vi "RP proccess data.vi"() -> ()   [LabVIEW 2015]
uses:
  <vilib>/Analysis/NI_AALPro.lvlib
panel:
  in  "Filed tiime shift":dbl format="%#_6p"
  out "Phase":dbl
  out "Waveform Graph 2":waveform(dbl)(graph)
  in  "Clip units of Ts off":dbl
  in  "Filter type":enum16{"None", "IIR", "FIR"}(ring)=enum."FIR"
  in  "Save output":bool
  in  "Phase shift":dbl step=90.0
  in  "Integrate Bdot":bool
  in  "Fix time delay":bool=TRUE
  in  "Time constant":dbl=0.0001 format="%#_6p"
  out "XY Graph":cluster{dbl[], "Y":dbl[]}[](graph)
  out "Error Out":errorcluster
  in  "Bdot calibration":dbl=2506.0
  in  "offset length":i32=990000
  out "Waveform Graph":waveform(dbl)[](graph)
  in  "Bdot channel":string="Field_fixed"
  in  "Signal channel":string="CH0"
  in  "Bdot file":path
  in  "Signal file":path
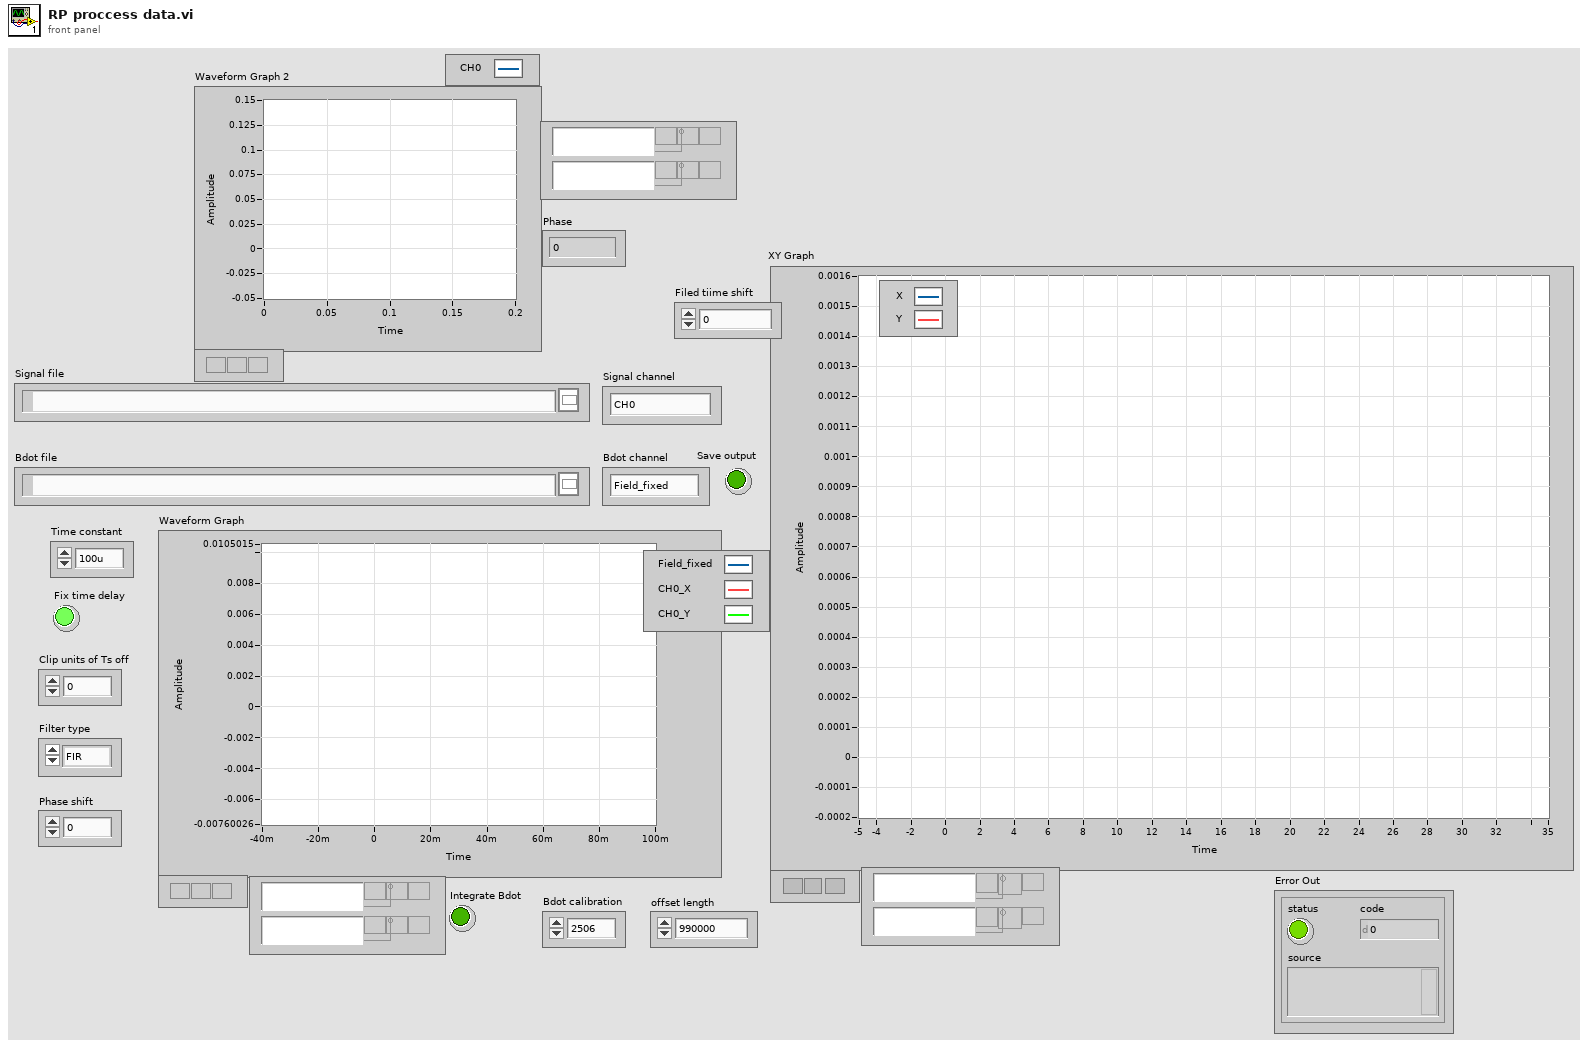
[diagram p1: front panel]
types:
  T1 = enum16{"open", "open or create", "create or replace", "create", "open (read-only)"}
  T2 = cluster{"Waveform":waveform(dbl), "Waveform":waveform(dbl)}
  T3 = cluster{"Waveform":waveform(dbl), "Waveform":waveform(dbl)}[]
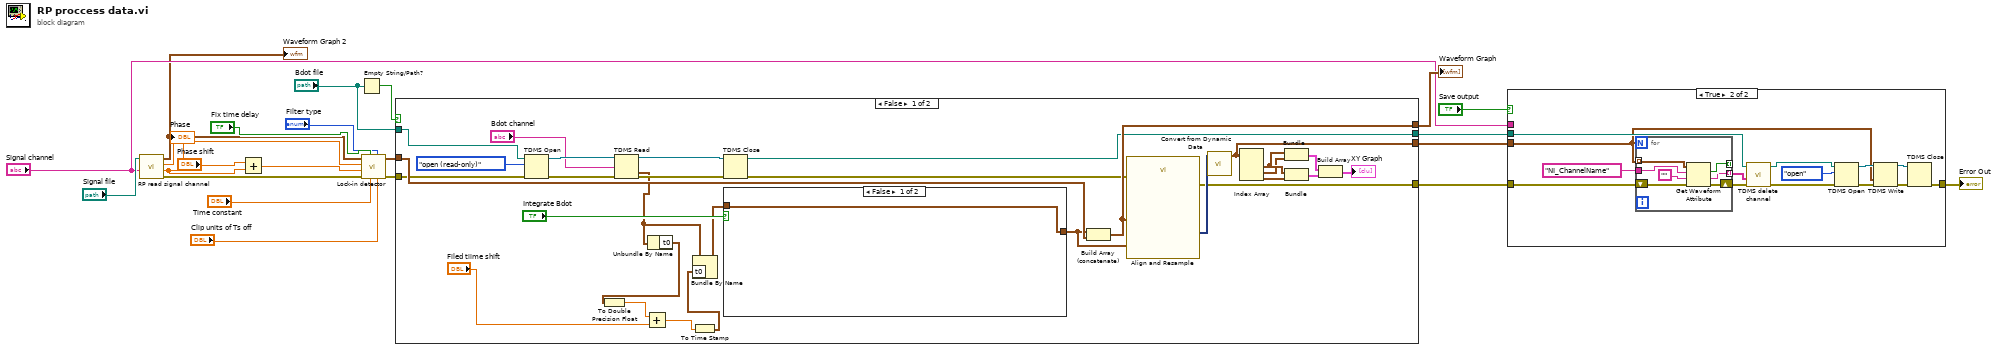
[diagram p0: block diagram]
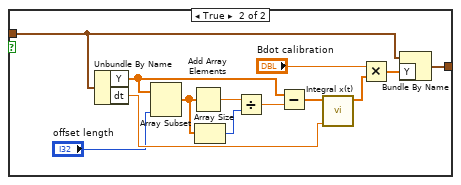
[diagram p2: hidden frame]
diagram:
  n1 = call "RP read signal channel.vi"("Channel name"="Signal channel", "File"="Signal file") -> ("Error Out"=w19:errorcluster, "Phase"=w20:dbl, "Frequency"=w21:dbl, "Data out"=w1:waveform(dbl))  [unwired: 3 in, 3 out]
  "Waveform Graph 2" <- w1
  "Phase" <- w20
  n2 = Add(x="Phase shift", y=w20) -> (x+y=w14:dbl)
  n3 = Empty String/Path?(string/path="Bdot file") -> (empty?=w4:bool)
  n4 = call "Lock-in detector.vi"("Clip units of Ts off"="Clip units of Ts off", "Filter type"="Filter type", "Time constant"="Time constant", "Fix time delay"="Fix time delay", "Error In"=w19, "Phase"=w14, "Frequency"=w21, "Data in"=w1) -> ("Error Out"=w3:errorcluster, "Data out"=w16:waveform(dbl)[])  [unwired: 2 in]
  n5 = case shown="False" w4 {
    tunnel: w16 -> [w45 w69]
    tunnel: [w38 w69] -> w15
    tunnel: [w37 w68] -> w11
    tunnel: [w34 w69] -> w8
    tunnel: "Bdot file" -> [w33 w68]
    tunnel: w3 -> [w30 w67]
    tunnel: [w31 w67] -> w2
    frame False {
      n6 = TDMS Open(8:w30, 10:T1."open (read-only)" ("operation (0:open)"), 11:w33) -> (0:w51:errorcluster, 3:w50:refnum<k34>)  [unwired: 4 in]
      n7 = TDMS Read(0:w50, 7:"Bdot channel", 11:w51) -> (4:w47:refnum<k34>, 10:w24:waveform(dbl), 15:w48:errorcluster)  [unwired: 5 in, 3 out]
      n8 = Unbundle By Name(w24) -> ("t0"=w29:timestamp)
      n9 = To Double Precision Float(number=w29) -> (double precision float=w28:dbl)
      n10 = Add(x=w28, y="Filed tiime shift") -> (x+y=w26:dbl)
      n11 = To Time Stamp(1:w26) -> (0:w25:timestamp)
      n12 = Bundle By Name(cluster=w24, "t0"=w25) -> (w23:waveform(dbl))
      n13 = TDMS Close(8:w48, 11:w47) -> (0:w32:errorcluster, 3:w37:path)
      n14 = case shown="False" "Integrate Bdot" {
        tunnel: w23 -> [w53 w56]
        tunnel: [w53 w54] -> w44
        frame False {
        }
        frame True {
          n15 = Unbundle By Name(w56) -> ("Y"=w59:dbl[], "dt"=w66:dbl)
          n16 = Array Subset(array=w59, length="offset length") -> (w63:dbl[])  [unwired: 1 in]
          n17 = Add Array Elements(numeric array=w63) -> (sum=w62:dbl)
          n18 = Array Size(array=w63) -> (size(s)=w61:i32)
          n19 = Divide(x=w62, y=w61) -> (x/y=w58:dbl)
          n20 = Subtract(x=w59, y=w58) -> (x-y=w60:dbl[])
          n21 = call <vilib>:"Integral x(t).vi"("dt"=w66, "X"=w60) -> ("Integral X"=w65:dbl[])  [unwired: 8 in, 1 out]
          n22 = Multiply(x="Bdot calibration", y=w65) -> (x*y=w55:dbl[])
          n23 = Bundle By Name(cluster=w56, "Y"=w55) -> (w54:waveform(dbl))
        }
      }
      n24 = Build Array (concatenate)(w44, w45) -> (w38:waveform(dbl)[])
      n25 = call "Align and Resample"("Reference Signal"=w44, "error in (no error)"=w32, "Signals"=w38) -> ("error out"=w31:errorcluster, "Resampled Signals"=w43:dynamicdata)  [unwired: 6 in, 1 out]
      n26 = call "Convert from Dynamic Data"("Dynamic Data Type"=w43) -> ("Array of Waveform"=w34:waveform(dbl)[])  [unwired: 3 in]
      n27 = Index Array(array=w34) -> (element #1=w42:waveform(dbl), element #2=w36:waveform(dbl), element #3=w35:waveform(dbl))  [unwired: 3 in]
      n28 = Bundle("Waveform"=w42, "Waveform"=w36) -> (w41:T2)  [unwired: 1 in]
      n29 = Bundle("Waveform"=w42, "Waveform"=w35) -> (w40:T2)  [unwired: 1 in]
      n30 = Build Array(w41, w40) -> (→"XY Graph":T3)
    }
    frame True {
    }
  }
  "Waveform Graph" <- w15
  n31 = case shown="True" "Save output" {
    tunnel: w11 -> [_ w80]
    tunnel: w2 -> [w70 w74]
    tunnel: [w70 w82] -> w10
    tunnel: "Signal channel" -> [_ _]
    tunnel: w8 -> [_ w71]
    frame False {
    }
    frame True {
      n32 = for {
        tunnel: w71 -> [w91] mode=indexing
        tunnel: "NI_ChannelName" ("name") -> [w90]
        tunnel: [w89] -> _ mode=indexing
        tunnel: [w85] -> w72 mode=indexing
        shift-right: [w87] -> w73
        shift-left: w74 -> [w88]
        n33 = Get Waveform Attribute(4:w88, 5:"", 6:w90, 7:w91) -> (0:w87:errorcluster, 1:w85:string, 2:w89:bool)  [unwired: 1 out]
      }
      n34 = call "TDMS delete channel.vi"("error in (no error)"=w73, "Channels"=w72, "file path"=w80) -> ("error out"=w79:errorcluster, "file path out"=w78:path)  [unwired: 6 in, 1 out]
      n35 = TDMS Open(8:w79, 10:T1."open" ("operation (0:open)"), 11:w78) -> (0:w76:errorcluster, 3:w77:refnum<k34>)  [unwired: 4 in]
      n36 = TDMS Write(0:w77, 9:w71, 11:w76) -> (4:w84:refnum<k34>, 15:w83:errorcluster)  [unwired: 3 in, 2 out]
      n37 = TDMS Close(8:w83, 11:w84) -> (0:w82:errorcluster)  [unwired: 1 out]
    }
  }
  "Error Out" <- w10
